vi "get 9V monitor voltage.vi"(8 "error in (no error)":errorcluster, 9 "Descriptions":string[](array[string]), 10 "Array":string[](array[string]), 11 "Array 2":refnum<k24>[](array[refnum])) -> (0 "error out":errorcluster, 3 "9V Voltage Monitor":dbl)   [LabVIEW 2016]
uses:
  C:/Program Files (x86)/National Instruments/LabVIEW 2016/vi.lib/ULx/ULx_LV.dll
  <vilib>/Analysis/baseanly.llb/Mean (DBL).vi
  <vilib>/ULx/Read.llb/ULx Read (Analog 1D DBL 1Chan NSamp).vi
  <vilib>/Analysis/NI_AALBase.lvlib
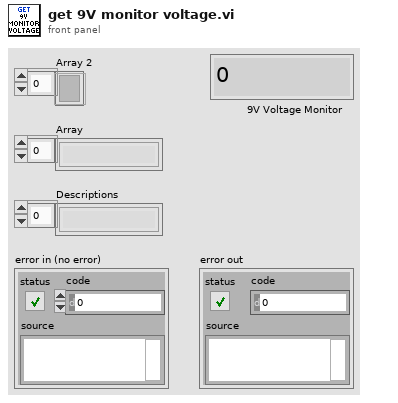
[diagram p1: front panel]
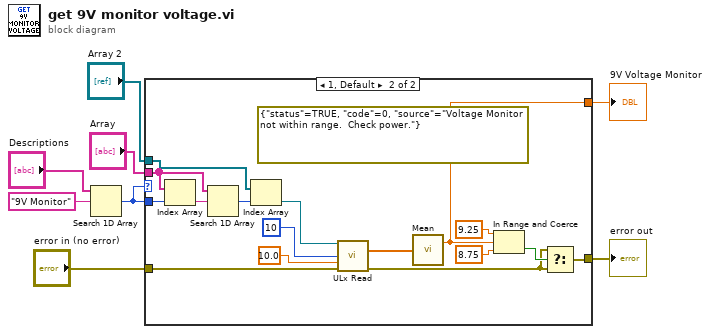
[diagram p0: block diagram]
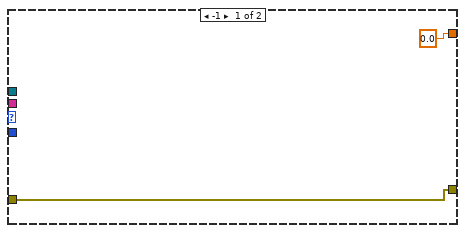
[diagram p2: hidden frame]
diagram:
  n1 = Search 1D Array(1D array="Descriptions", element="9V Monitor") -> (index of element=w3:i32)  [unwired: 1 in]
  n2 = case shown="1, Default" w3 {
    tunnel: "Array 2" -> [_ w26]
    tunnel: w3 -> [_ w20]
    tunnel: "error in (no error)" -> [w10 w24]
    tunnel: [w10 w13] -> w5
    tunnel: "Array" -> [_ w18]
    tunnel: [0.0 ("mean") w12] -> w8
    frame -1 {
    }
    frame 1, Default {
      (unwired) errorcluster {"status"=TRUE, "code"=0, "source"="Voltage Monitor not within range.  Check power."} ("t")
      n3 = Index Array(array=w18, index=w20) -> (element=w19:string)
      n4 = Search 1D Array(1D array=w18, element=w19) -> (index of element=w17:i32)  [unwired: 1 in]
      n5 = Index Array(array=w26, index=w17) -> (element=w25:refnum<k24>)
      n6 = call-poly <vilib>:"ULx Read.vi"("task in"=w25, "number of samples per channel"=10, "timeout"=10.0, "error in"=w24) -> ("data"=w21:dbl[], "error out"=w11:errorcluster)  [unwired: 9 in, 1 out]
      n7 = call-poly <vilib>:"Mean.vi"("X"=w21) -> ("mean"=w12:dbl)  [unwired: 1 out]
      n8 = In Range and Coerce(upper limit=9.25, x=w12, lower limit=8.75) -> (In Range?=w14:bool)  [unwired: 1 out]
      n9 = Select(t=w11, s=w14, f=w11) -> (s? t:f=w13:errorcluster)
    }
  }
  "9V Voltage Monitor" <- w8
  "error out" <- w5
